vi "Create Command.vi"(10 "Command Queue":refnum<queue>) -> (3 "Initialize Application.lvclass":refnum<class "Initialize Application.lvclass">)   [LabVIEW 2010, in "Initialize Application.lvclass"]
doc: "This instance of Create Command.vi writes the value of the Command Queue reference to the data stored within Initialize Application.lvclass."
uses:
  Initialize Application.lvclass
  Application Command/Application Command.lvclass
  Initialize Application.lvclass/Initialize Application.ctl
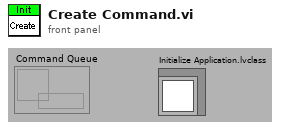
[diagram p1: front panel]
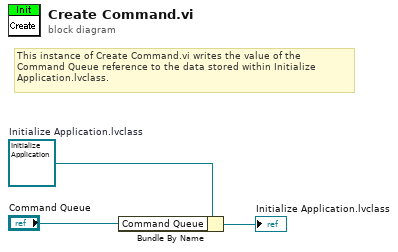
[diagram p0: block diagram]
diagram:
  w3 = refnum<class "Initialize Application.lvclass"> refnum  # Initialize Application.lvclass
  # "This instance of Create Command.vi writes the value of the  Command Queue reference to the data stored within Initialize Application.lvclass."
  n1 = Bundle By Name "Bundle By Name"(cluster=w3, "Command Queue"="Command Queue") -> (→"Initialize Application.lvclass":refnum<class "Initialize Application.lvclass">)
